vi "Abort Motion.vi"(8 "error in (no error)":errorcluster, 11 "Gantry In":refnum<k24>) -> (0 "error out":errorcluster, 3 "Gantry Out":refnum<k24>)   [LabVIEW 2020, in "A3200.lvclass"]
uses:
  A3200.lvclass
  C:/Program Files (x86)/Aerotech/A3200/LabVIEW/2010/Bin/Aerotech.A3200.dll
  Program Files (x86)/Aerotech/A3200/LabVIEW/2010/Bin/Aerotech.A3200.dll
  Drivers/Aerotech A3200/Aerotech VIs.lvlib
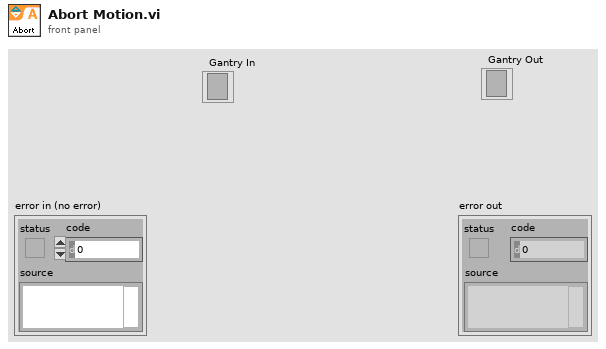
[diagram p1: front panel]
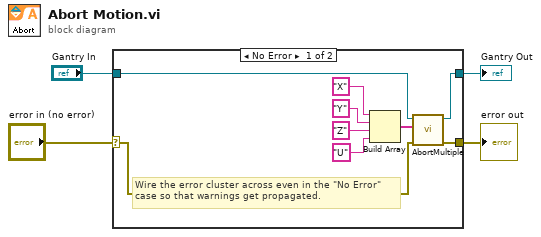
[diagram p0: block diagram]
diagram:
  n1 = case shown="No Error" "error in (no error)" {
    selector: "error in (no error)" -> [w6 w15]
    tunnel: [w5 w15] -> w3
    tunnel: "Gantry In" -> [w8 w14]
    tunnel: [w7 w14] -> w1
    frame No Error {
      # "Wire the error cluster across even in the \"No Error\"\ncase so that warnings get propagated."
      n2 = Build Array("X", "Y", "Z", "U") -> (w9:string[])
      n3 = call "AbortMultiple.vi"("error in (no error)"=w6, "axis names"=w9, "controller in"=w8) -> ("error out"=w5:errorcluster, "controller out"=w7:refnum<k24>)  [unwired: 7 in]
    }
    frame Error {
    }
  }
  "error out" <- w3
  "Gantry Out" <- w1
